vi "VISA Connection Start.vi"(6 "Error In":errorcluster, 7 "Ports to search":i32=25, 8 "Markers":T1, 9 "Baud":i32=9600) -> (0 "Error Out":errorcluster, 2 "Found?":bool, 3 "VISA resource name":refnum<visa-resource-name>)   [LabVIEW 2014, in "VISA Connection Template.lvlib"]
uses:
  VISA Connection Template.lvlib
  <vilib>/Instr/_visa.llb/VISA Configure Serial Port (Instr).vi
  <vilib>/Instr/_visa.llb/Select Event Type.ctl
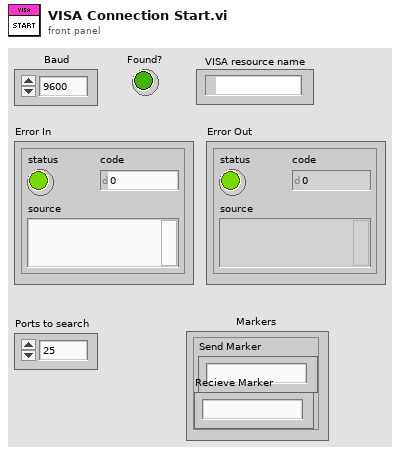
[diagram p1: front panel]
types:
  T1 = cluster{"Send Marker":string, "Recieve Marker":string}
  T2 = typedef "Select Event Type.ctl" = u32
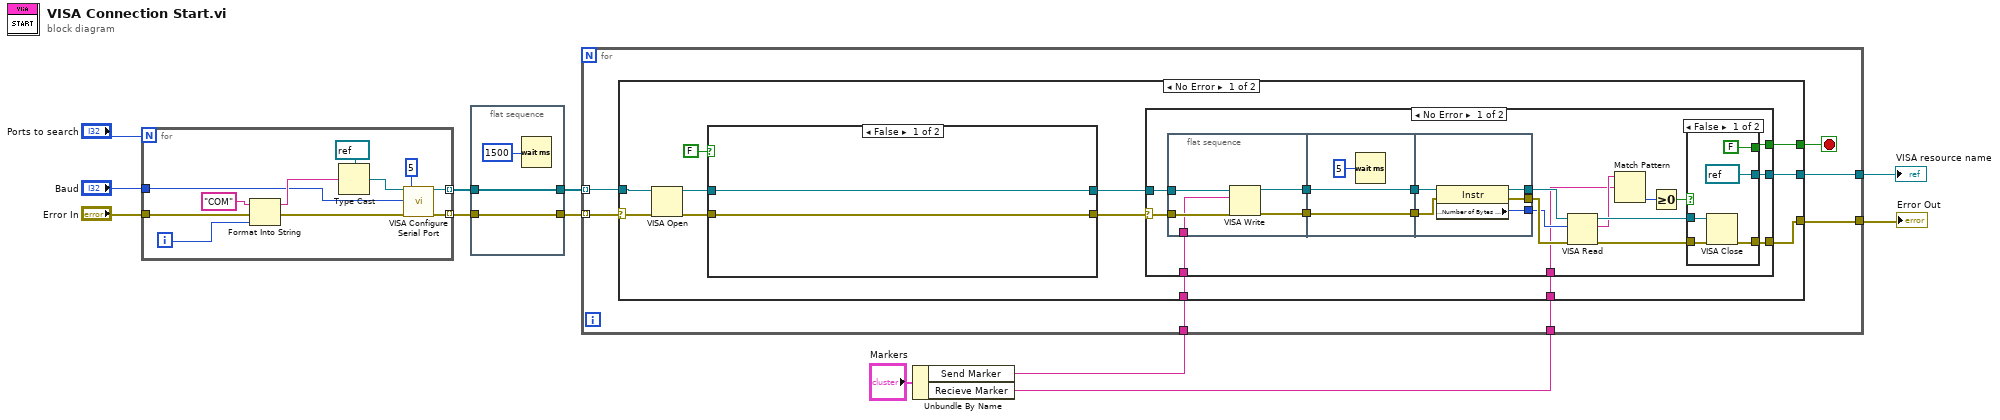
[diagram p0: block diagram]
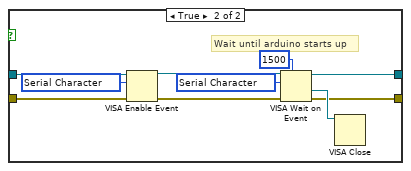
[diagram p2: hidden frame]
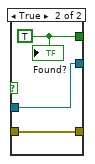
[diagram p3: hidden frame]
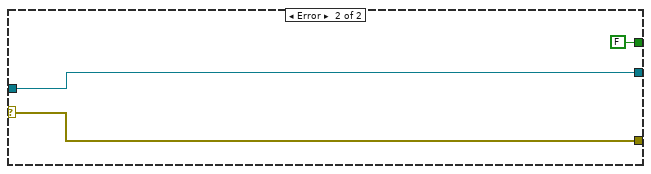
[diagram p4: hidden frame]
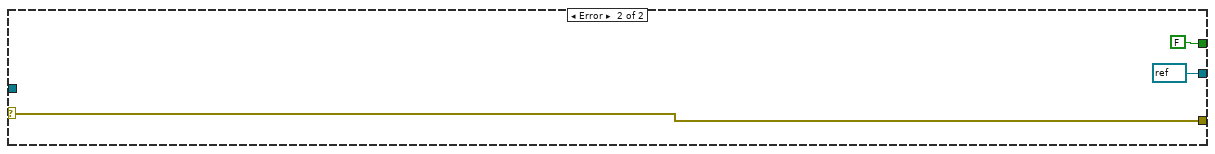
[diagram p5: hidden frame]
diagram:
  n1 = for {
    N: "Ports to search" -> [_]
    tunnel: "Error In" -> [w16]
    tunnel: "Baud" -> [w15]
    tunnel: [w14] -> w8 mode=indexing
    tunnel: [w13] -> w7 mode=indexing
    i -> [w17]
    n2 = Format Into String(initial string="COM", error in=w16, w17) -> (resulting string=w20:string, error out=w23:errorcluster)  [unwired: 1 in]
    n3 = Type Cast(type=refnum<visa-resource-name> refnum ("portVisa"), x=w20) -> (*(type *) &x=w22:refnum<visa-resource-name>)
    n4 = call-poly "VISA Configure Serial Port"("VISA resource name"=w22, "timeout (10sec)"=u32 5, "baud rate (9600)"=w15, "error in (no error)"=w23) -> ("VISA resource name out"=w14:refnum<visa-resource-name>, "error out"=w13:errorcluster)  [unwired: 10 in]
  }
  n5 = flat-sequence {
    tunnel: w8 -> [w26]
    tunnel: w7 -> [w25]
    tunnel: [w26] -> w6
    tunnel: [w25] -> w5
    frame #0 {
      n6 = Wait (ms)(milliseconds to wait=u32 1500) -> ()  [unwired: 1 out]
    }
  }
  n7 = Unbundle By Name("Markers") -> ("Send Marker"=w3:string, "Recieve Marker"=w2:string)
  n8 = for {
    tunnel: [w32] -> w11
    tunnel: [w31] -> w12
    tunnel: w6 -> [w30] mode=indexing
    tunnel: w5 -> [w29] mode=indexing
    tunnel: w3 -> [w28]
    tunnel: w2 -> [w27]
    stop <- w33 stop-if-true
    n9 = case shown="No Error" w29 {
      selector: w29 -> [w42 w102]
      tunnel: w30 -> [w44 _]
      tunnel: [w45 FALSE] -> w33
      tunnel: [w41 w102] -> w31
      tunnel: [w40 refnum<visa-resource-name> refnum ("VISA resource name out")] -> w32
      tunnel: w28 -> [w35 _]
      tunnel: w27 -> [w34 _]
      frame No Error {
        n10 = VISA Open(error in (no error)=w42, VISA resource name=w44) -> (VISA resource name=w43:refnum<visa-resource-name>, error out=w39:errorcluster)  [unwired: 3 in]
        n11 = case shown="False" FALSE {
          tunnel: w43 -> [w47 w57]
          tunnel: w39 -> [w46 w56]
          tunnel: [w47 w52] -> w38
          tunnel: [w46 w48] -> w37
          frame False {
          }
          frame True {
            w51 = T2 1073684533 items=["Service Request"=1073684491, "Trigger"=3221168138, "Clear"=1073684493, "VXI Signal"=1073684512, "VXI/VME Interrupt"=3221168161, "VXI/VME Sysfail"=1073684509, "VXI/VME Sysreset"=1073684510, "GPIB CIC"=1073684498, "GPIB Talk"=1073684499, "GPIB Listen"=1073684500, "PXI Interrupt"=1073684514, "Serial Break"=1073684515, "Serial TermChar"=1073684516, "Serial CTS"=1073684521, "Serial DSR"=1073684522, "Serial DCD"=1073684524, "Serial RI"=1073684526, "Serial Character"=1073684533, "USB Interrupt"=1073684535, "All Enabled"=1073709055] ("Event Type")
            w55 = T2 1073684533 items=["Service Request"=1073684491, "Trigger"=3221168138, "Clear"=1073684493, "VXI Signal"=1073684512, "VXI/VME Interrupt"=3221168161, "VXI/VME Sysfail"=1073684509, "VXI/VME Sysreset"=1073684510, "GPIB CIC"=1073684498, "GPIB Talk"=1073684499, "GPIB Listen"=1073684500, "PXI Interrupt"=1073684514, "Serial Break"=1073684515, "Serial TermChar"=1073684516, "Serial CTS"=1073684521, "Serial DSR"=1073684522, "Serial DCD"=1073684524, "Serial RI"=1073684526, "Serial Character"=1073684533, "USB Interrupt"=1073684535, "All Enabled"=1073709055] ("Event Type")
            # "Wait until arduino starts up"
            n12 = VISA Enable Event(8:w56, 10:w55, 11:w57) -> (0:w53:errorcluster, 3:w54:refnum<visa-resource-name>)  [unwired: 1 in]
            n13 = VISA Wait on Event(7:u32 1500 ("timeout (0)"), 8:w53, 10:w51, 11:w54) -> (0:w48:errorcluster, 1:w49:refnum<visa-resource-name>, 3:w52:refnum<visa-resource-name>)  [unwired: 1 in, 1 out]
            n14 = VISA Close(VISA resource name=w49) -> ()  [unwired: 1 in, 1 out]
          }
        }
        n15 = case shown="No Error" w37 {
          selector: w37 -> [w64 w99]
          tunnel: [w75 FALSE] -> w45
          tunnel: [w70 w99] -> w41
          tunnel: [w69 w98] -> w40
          tunnel: w38 -> [w68 w98]
          tunnel: w35 -> [w63 _]
          tunnel: w34 -> [w62 _]
          frame No Error {
            n16 = flat-sequence {
              tunnel: [w81] -> w61
              tunnel: [w80] -> w59
              tunnel: w64 -> [w79]
              tunnel: w68 -> [w78]
              tunnel: w63 -> [w77]
              tunnel: w61 -> [w84]
              tunnel: [w84] -> w60
              tunnel: w59 -> [w83]
              tunnel: [w83] -> w58
              tunnel: w60 -> [w89]
              tunnel: w58 -> [w88]
              tunnel: [w87] -> w65
              tunnel: [w86] -> w67
              tunnel: [w85] -> w66
              frame #0 {
                n17 = VISA Write(VISA resource name=w78, write buffer=w77, error in (no error)=w79) -> (VISA resource name out=w81:refnum<visa-resource-name>, error out=w80:errorcluster)  [unwired: 1 out]
              }
              frame #1 {
                n18 = Wait (ms)(milliseconds to wait=u32 5) -> ()  [unwired: 1 out]
              }
              frame #2 {
                n19 = property class="Instr"(reference=w89, error in=w88) -> (reference out=w85:refnum<visa-resource-name>, error out=w86:errorcluster, "Serial Settings:Number of Bytes at Serial Port"=w87:u32)
              }
            }
            n20 = VISA Read(VISA resource name=w66, byte count=w65, error in (no error)=w67) -> (VISA resource name out=w76:refnum<visa-resource-name>, read buffer=w74:string, error out=w71:errorcluster)  [unwired: 1 out]
            n21 = Match Pattern(string=w74, regular expression=w62) -> (offset past match=w73:i32)  [unwired: 1 in, 3 out]
            n22 = Greater Or Equal To 0?(x=w73) -> (x >= 0?=w72:bool)
            n23 = case shown="False" w72 {
              tunnel: w76 -> [w93 w96]
              tunnel: [FALSE w95] -> w75
              tunnel: w71 -> [w92 w97]
              tunnel: [w91 w97] -> w70
              tunnel: [refnum<visa-resource-name> refnum ("VISA resource name out") w96] -> w69
              frame False {
                n24 = VISA Close(VISA resource name=w93, error in (no error)=w92) -> (error out=w91:errorcluster)
              }
              frame True {
                w95 = TRUE
                "Found?" <- w95
              }
            }
          }
          frame Error {
          }
        }
      }
      frame Error {
      }
    }
  }
  "Error Out" <- w12
  "VISA resource name" <- w11
